vi "Connection_GET.vi"(8 "error in":errorcluster, 11 "server in":refnum<class "RT FlexRIO Server TCP.lvclass">) -> (0 "error out":errorcluster, 2 "connection":refnum<k5>, 3 "server out":refnum<class "RT FlexRIO Server TCP.lvclass">)   [LabVIEW 2017, in "RT FlexRIO Server TCP.lvclass"]
uses:
  RT FlexRIO Server TCP.lvclass
  RT FlexRIO Server TCP.lvclass/RT FlexRIO Server TCP.ctl
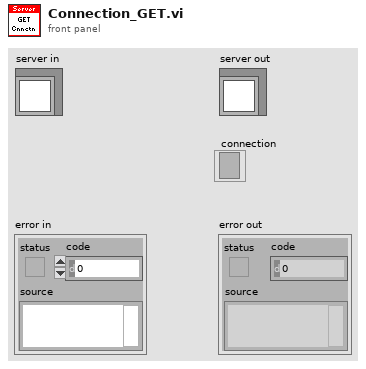
[diagram p1: front panel]
types:
  T1 = typedef "RT FlexRIO Server TCP.lvclass/SessionData.ctl" = cluster{"listener":refnum<k5>, "connection":refnum<k5>, "state":T2, "incoming":refnum<queue>, "outgoing":refnum<queue>, "state request":refnum<user-event>, "state changed":refnum<user-event>}
  T2 = typedef "RT FlexRIO Server TCP.lvclass/connection state.ctl" = enum16{"started", "connected", "stopped"}
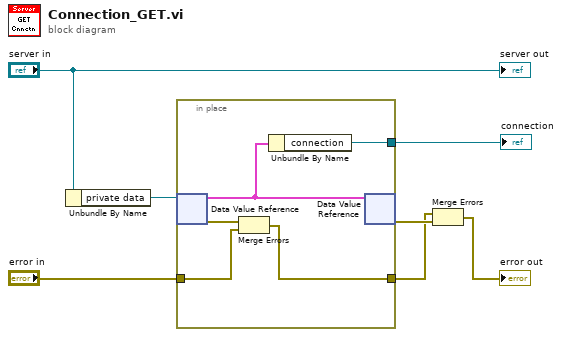
[diagram p0: block diagram]
diagram:
  n1 = Unbundle By Name("server in") -> ("private data"=w7:refnum<data-value>)
  n2 = in-place {
    in-place-border: "error in" -> [w11]
    in-place-border: [w10] -> w4
    in-place-border: [w8] -> w1
    n3 = in-place-dvr #1(w7) -> (w9:T1, w12:errorcluster)
    n4 = Merge Errors(w12, w11) -> (w10:errorcluster)
    n5 = Unbundle By Name(w9) -> ("connection"=w8:refnum<k5>)
    n6 = in-place-dvr #1(w9) -> (w5:errorcluster)  [unwired: 1 out]
  }
  "connection" <- w1
  n7 = Merge Errors(w4, w5) -> (→"error out":errorcluster)
  "server out" <- "server in"
